vi "CAN service.vi"(4 "error in (no error)":errorcluster, 5 "Data":u8[](array[numeric]), 6 "COB id":i32, 7 "CANopen in":refnum<class "CANopen.lvclass">) -> (0 "error out":errorcluster, 2 "Processed?":bool, 3 "CANopen out":refnum<class "CANopen.lvclass">)   [LabVIEW 2017, in "canopen.lvlib" / "CANopen.lvclass"]
doc: "Tries to store the data of a COB (usually an SDO message) into a specific variable. The correct COB-ID must be present inside the provided \"Map\", usually esplicitely requested as a response to an \"SDO upload\". The implementation is quite similar to the PDO handling provided by \"CAN process\", with the notable difference that in this case the entries in the map are consumed."
uses:
  CANopen.lvclass
  CANopen.lvclass/CANopen.ctl
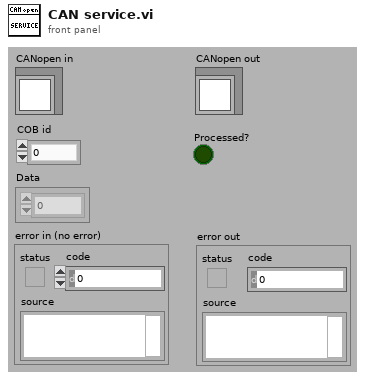
[diagram p1: front panel]
types:
  T1 = cluster{"CobID":u32, "Data offset":u8, "Data size":u8, "Destination":refnum<vi>}[]
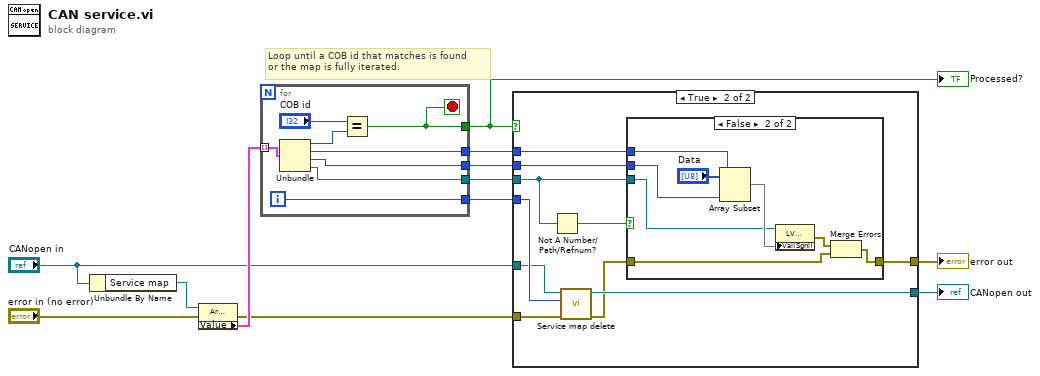
[diagram p0: block diagram]
diagram:
  # "Loop until a COB id that matches is found\nor the map is fully iterated."
  n1 = Unbundle By Name("CANopen in") -> ("Service map"=w4:refnum<vi>)
  n2 = property class="Arr (strict)"(reference=w4, error in="error in (no error)") -> (error out=w8:errorcluster, "Value"=w10:T1)  [unwired: 1 out]
  n3 = for {
    tunnel: w10 -> [w20] mode=indexing
    tunnel: [w18] -> w12
    tunnel: [w17] -> w11
    tunnel: [w15] -> w3
    tunnel: [w14] -> w2
    tunnel: [w13] -> w1
    i -> [w17]
    stop <- w18 stop-if-true
    n4 = Unbundle(w20) -> ("CobID"=w19:u32, "Data offset"=w13:u8, "Data size"=w15:u8, "Destination"=w14:refnum<vi>)
    n5 = Equal?(x="COB id", y=w19) -> (x = y?=w18:bool)
  }
  "Processed?" <- w12
  n6 = case shown="True" w12 {
    tunnel: w11 -> [_ w31]
    tunnel: w8 -> [w22 w32]
    tunnel: [w22 w24] -> w7
    tunnel: [w21 w30] -> w6
    tunnel: "CANopen in" -> [w21 w29]
    tunnel: w3 -> [_ w27]
    tunnel: w2 -> [_ w25]
    tunnel: w1 -> [_ w28]
    frame False {
    }
    frame True {
      n7 = Not A Number/Path/Refnum?(number/path/refnum=w25) -> (NaN/Path/Refnum?=w26:bool)
      n8 = call "Service map delete.vi"("error in (no error)"=w32, "Index"=w31, "CANopen in"=w29) -> ("error out"=w23:errorcluster, "CANopen out"=w30:refnum<class "CANopen.lvclass">)  [unwired: 3 out]
      n9 = case shown="False" w26 {
        tunnel: [w33 w37] -> w24
        tunnel: w28 -> [_ w40]
        tunnel: w27 -> [_ w39]
        tunnel: w25 -> [_ w34]
        tunnel: w23 -> [w33 w36]
        frame True {
        }
        frame False {
          n10 = Array Subset(array="Data", index=w40, length=w39) -> (w35:u8[])
          n11 = property class="LVVar"(reference=w34, "Val(Sgnl)"=w35) -> (error out=w38:errorcluster)  [unwired: 1 in, 1 out]
          n12 = Merge Errors(w38, w36) -> (w37:errorcluster)
        }
      }
    }
  }
  "error out" <- w7
  "CANopen out" <- w6
